vi "Send Auto Probe Sense Value [PAS].vi"(7 "Message Priority (Normal)":T1=enum."Normal", 8 "error in (no error)":errorcluster, 10 "channel name (\"CHANNEL1\")":string="CHANNEL1", 11 "Message Enqueuer":refnum<class "Message Enqueuer.lvclass">) -> (0 "error out":errorcluster, 3 "Message Enqueuer out":refnum<class "Message Enqueuer.lvclass">)   [LabVIEW 2015, in "CS++Scope.lvlib" / "Auto Probe Sense Value [PAS] Msg.lvclass"]
doc: "Sends the <B>CS++Scope.lvlib:Auto Probe Sense Value [PAS] Msg.lvclass</B> message.\n\n<B>CS++Scope.lvlib:CS++Scope.lvclass:Auto Probe Sense Value [PAS].vi</B> Description:\n\nThe VI returns the probe attenuation value the oscilloscope senses. You enable the automatic probe sense capability by setting the Probe Attenuation parameter of the IviScope Configure Channel VI to IVISCOPE_VAL_PROBE_SENSE_ON (-1).\n\nNote\n\n If you disable the automatic probe sense capability, this VI returns the manual probe attenuation setting."
uses:
  Auto Probe Sense Value [PAS] Msg.lvclass
  <vilib>/ActorFramework/Message Enqueuer/Message Enqueuer.lvclass
  <vilib>/ActorFramework/Message Enqueuer/Message Priority.ctl
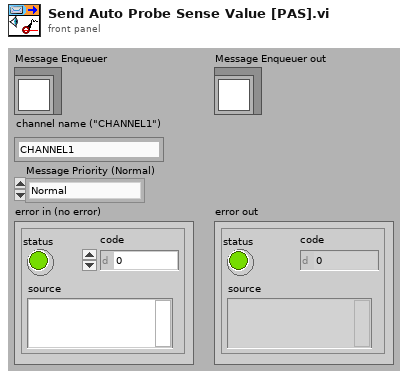
[diagram p1: front panel]
types:
  T1 = typedef "Actor Framework.lvlib/Message Enqueuer.lvclass/Message Priority.ctl" = enum16{"Low", "Normal", "High"}
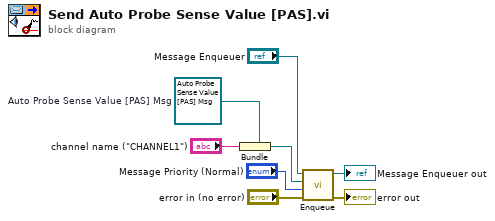
[diagram p0: block diagram]
diagram:
  w2 = refnum<class "Auto Probe Sense Value [PAS] Msg.lvclass"> refnum  # Auto Probe Sense Value [PAS] Msg
  n1 = Bundle(cluster=w2, "channel name (\"CHANNEL1\")") -> (w5:refnum<class "Auto Probe Sense Value [PAS] Msg.lvclass">)
  n2 = call <vilib>:"Enqueue.vi"("error in (no error)"="error in (no error)", "Message Priority (Normal)"="Message Priority (Normal)", "Message"=w5, "Message Enqueuer in"="Message Enqueuer") -> ("error out"=→"error out":errorcluster, "Message Enqueuer out"=→"Message Enqueuer out":refnum<class "Message Enqueuer.lvclass">)  [unwired: 6 in]
